vi "File Upload Throughput.vi"() -> ()   [LabVIEW 2019]
uses:
  <vilib>/Skyline/Configuration/Configuration HTTP_class/NI Skyline Configuration HTTP.lvclass/NI Skyline Configuration HTTP.ctl
  <vilib>/Skyline/Configuration/Configuration HTTP_class/Open Configuration HTTP Auto.vi
  <vilib>/Skyline/Configuration/HTTP/Open Configuration Auto (Custom).vi
  <vilib>/Skyline/File/HTTP/NI Skyline File HTTP.lvclass
  C:/Program Files (x86)/National Instruments/LabVIEW 2019/vi.lib/Skyline/File/Base/NI Skyline File Base.lvclass
  <vilib>/Skyline/Configuration/HTTP/Configuration File Cache.vi
  <vilib>/Skyline/Configuration/HTTP/Initialize From Auto Configuration.vi
  <vilib>/Skyline/File/HTTP/Send File HTTP.vi
  <vilib>/Skyline/File/HTTP/Open File HTTP.vi
  <vilib>/Skyline/File/File/Delete (Single).vi
  <vilib>/Skyline/Configuration/Configuration HTTP_class/NI Skyline Configuration HTTP.lvclass
  <vilib>/Skyline/File/File/NI Skyline File.lvclass
  <vilib>/Skyline/File/Base/NI Skyline File Base.lvclass
  <vilib>/Skyline/Configuration/Configuration_class/NI Skyline Configuration.lvclass
panel:
  out "Throughput (B/S)":dbl format="%#.2p"
  out "Total Time (Seconds)":dbl
  out "Total Bytes Sent":i64 format="%.2p"
  out "Files Deleted":u32
  out "Time to Send File":u32(graph)
  out "File Size (Bytes)":i64 format="%.2p"
  out "Files Sent":u32
  in  "Stop":bool
  in  "Test Duration (Seconds)":dbl=3600.0
  in  "File Path Control":path
  out "Time to Send File (mS)":u32
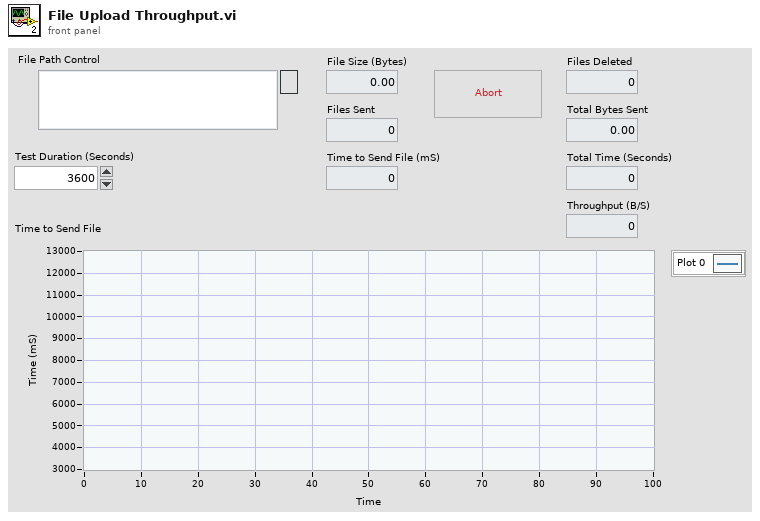
[diagram p1: front panel]
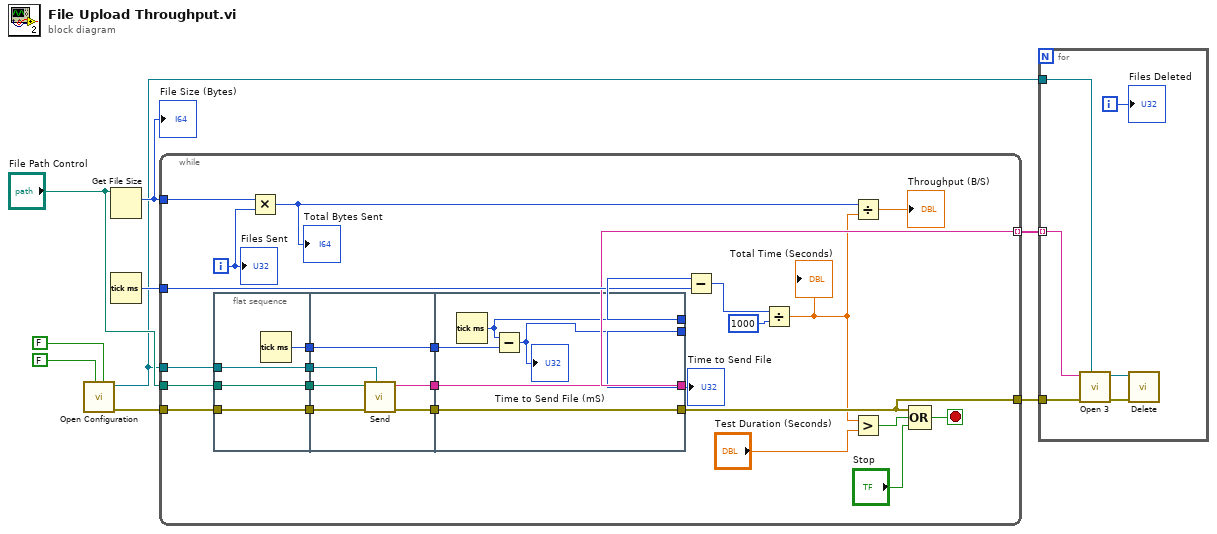
[diagram p0: block diagram]
diagram:
  n1 = call-poly <vilib>:"Open Configuration.vi"("HTTPS only?"=FALSE, "verify server?"=FALSE) -> ("error out"=w5:errorcluster, "configuration"=w4:refnum<class "NI Skyline Configuration HTTP.lvclass">)  [unwired: 8 in]
  n2 = Get File Size(file="File Path Control") -> (size (in bytes)=w6:i64)  [unwired: 1 in, 2 out]
  "File Size (Bytes)" <- w6
  n3 = Tick Count (ms)() -> (millisecond timer value=w9:u32)
  n4 = while {
    tunnel: w9 -> [w32]
    tunnel: "File Path Control" -> [w14]
    tunnel: [w28] -> w7 mode=indexing
    tunnel: w6 -> [w24]
    tunnel: w4 -> [w17]
    tunnel: w5 -> [w15]
    tunnel: [w12] -> w3
    i -> [w25]
    stop <- w29 stop-if-true
    n5 = flat-sequence {
      tunnel: [w39] -> w35
      tunnel: [w38] -> w18
      tunnel: w17 -> [w38]
      tunnel: [w37] -> w16
      tunnel: w15 -> [w37]
      tunnel: w14 -> [w36]
      tunnel: [w36] -> w13
      tunnel: w35 -> [w45]
      tunnel: [w45] -> w34
      tunnel: [w44] -> w27
      tunnel: w18 -> [w43]
      tunnel: w16 -> [w42]
      tunnel: w13 -> [w41]
      tunnel: [w40] -> w11
      tunnel: w34 -> [w50]
      tunnel: [w49] -> w26
      tunnel: [w48] -> w33
      tunnel: [w47] -> w28
      tunnel: w27 -> [w47]
      tunnel: [w46] -> w12
      tunnel: w11 -> [w46]
      frame #0 {
        n6 = Tick Count (ms)() -> (millisecond timer value=w39:u32)
      }
      frame #1 {
        n7 = call-poly <vilib>:"Send.vi"("configuration"=w43, "error in (no error)"=w42, "path"=w41) -> ("error out"=w40:errorcluster, "id"=w44:string)  [unwired: 6 in]
      }
      frame #2 {
        n8 = Tick Count (ms)() -> (millisecond timer value=w48:u32)
        n9 = Subtract(x=w48, y=w50) -> (x-y=w49:u32)
        "Time to Send File (mS)" <- w49
      }
    }
    n10 = Multiply(x=w24, y=w25) -> (x*y=w23:i64)
    "Total Bytes Sent" <- w23
    n11 = Subtract(x=w33, y=w32) -> (x-y=w22:u32)
    n12 = Divide(x=w22, y=u32 1000) -> (x/y=w10:dbl)
    "Total Time (Seconds)" <- w10
    n13 = Divide(x=w23, y=w10) -> (x/y=→"Throughput (B/S)":dbl)
    n14 = Greater?(x=w10, y="Test Duration (Seconds)") -> (0:w31:bool)
    n15 = Compound Arithmetic op=OR(w12, w31, "Stop") -> (w29:bool)
    "Files Sent" <- w25
    "Time to Send File" <- w26
  }
  n16 = for {
    tunnel: w7 -> [w56] mode=indexing
    tunnel: w4 -> [w52]
    tunnel: w3 -> [w51]
    i -> [w53]
    n17 = call-poly <vilib>:"Open 3.vi"("configuration"=w52, "error in (no error)"=w51, "file id"=w56) -> ("error out"=w55:errorcluster, "file"=w54:refnum<class "NI Skyline File HTTP.lvclass">)  [unwired: 7 in]
    n18 = call-poly <vilib>:"Delete.vi"("error in (no error)"=w55, "file"=w54) -> ()  [unwired: 9 in, 1 out]
    "Files Deleted" <- w53
  }
